vi "Multi-Device Rx Streaming Time (Four Channels) (Host).vi"() -> ()   [LabVIEW 2021]
doc: "This template is for the Simple NI-USRP Streaming design, a design that shows the basics of streaming data from an NI 294x/295x device. Refer to the block diagram for more information about how to use this template."
uses:
  SubVIs/Start Trigger.ctl
  <vilib>/userdefined/Silver/nirio_resource_slv.ctl
  <vilib>/Utility/error.llb/DialogType.ctl
  <vilib>/measure/maspectr.llb/FFT Power Spectrum and PSD for 1 Chan (CDB).vi
  <vilib>/measure/NI_MAPro.lvlib
panel:
  in  "RIO Device 1":T1="RIO1"
  in  "RIO Device 0":T1="RIO0"
  in  "config tab":T2(tab)
  in  "device 0 rx config":T4={"transfer mode"=enum."Finite", "sample rate"=10000000.0, "number of samples"=8192, "start trigger"=enum."Immediate", "daughterboard 0 config"={"rf enable 0"=TRUE, "rf config 0"={"antenna"="RX1", "frequency"=5000000000.0, "gain"=40.0}, "rf enable 1"=TRUE, "rf config 1"={"antenna"="RX2", "frequency"=5000000000.0, "gain"=40.0}, "lo configuration"=enum."Shared"}, "daughterboard 1 config"={"rf enable 2"=TRUE, "rf config 2"={"antenna"="RX1", "frequency"=5000000000.0, "gain"=40.0}, "rf enable 3"=TRUE, "rf config 3"={"antenna"="RX2", "frequency"=5000000000.0, "gain"=40.0}, "lo configuration"=enum."Shared"}} {"daughterboard 1 config"."rf config 3"."gain" format="%#.1f"; "daughterboard 1 config"."rf config 3"."frequency" format="%#.3pHz"; "daughterboard 1 config"."rf config 2"."gain" format="%#.1f"; "daughterboard 1 config"."rf config 2"."frequency" format="%#.3pHz"; "daughterboard 0 config"."rf config 1"."gain" format="%#.1f"; "daughterboard 0 config"."rf config 1"."frequency" format="%#.3pHz"; "daughterboard 0 config"."rf config 0"."gain" format="%#.1f"; "daughterboard 0 config"."rf config 0"."frequency" format="%#.3pHz"; "sample rate" format="%#.3pS/s"}
  in  "device 1 rx config":T4={"transfer mode"=enum."Finite", "sample rate"=10000000.0, "number of samples"=8192, "start trigger"=enum."Immediate", "daughterboard 0 config"={"rf enable 0"=TRUE, "rf config 0"={"antenna"="RX1", "frequency"=5000000000.0, "gain"=40.0}, "rf enable 1"=TRUE, "rf config 1"={"antenna"="RX2", "frequency"=5000000000.0, "gain"=40.0}, "lo configuration"=enum."Shared"}, "daughterboard 1 config"={"rf enable 2"=TRUE, "rf config 2"={"antenna"="RX1", "frequency"=5000000000.0, "gain"=40.0}, "rf enable 3"=TRUE, "rf config 3"={"antenna"="RX2", "frequency"=5000000000.0, "gain"=40.0}, "lo configuration"=enum."Shared"}} {"daughterboard 1 config"."rf config 3"."gain" format="%#.1f"; "daughterboard 1 config"."rf config 3"."frequency" format="%#.3pHz"; "daughterboard 1 config"."rf config 2"."gain" format="%#.1f"; "daughterboard 1 config"."rf config 2"."frequency" format="%#.3pHz"; "daughterboard 0 config"."rf config 1"."gain" format="%#.1f"; "daughterboard 0 config"."rf config 1"."frequency" format="%#.3pHz"; "daughterboard 0 config"."rf config 0"."gain" format="%#.1f"; "daughterboard 0 config"."rf config 0"."frequency" format="%#.3pHz"; "sample rate" format="%#.3pS/s"}
  out "acquiring":bool caption="Acquiring"
  in  "reference frequency source":string(combo)="REF IN" caption="Reference Frequency Source"
  in  "indicator tab":T5(tab)
  out "power spectrum":cluster{"f0":dbl, "df":dbl, "magnitude":dbl[]}[](graph) caption="Power Spectrum"
  out "iq data":waveform(dbl)[](graph) caption="I & Q Data"
  out "rx.coerced config":T6(array[cluster]) caption="Coerced Configurations" {"channel 3"."sample rate" format="%#.3pS/s"; "channel 3"."gain" format="%#_1f"; "channel 3"."if2 lo" format="%#.3pHz"; "channel 3"."if1 lo" format="%#.3pHz"; "channel 3"."frequency" format="%#.3pHz"; "channel 2"."sample rate" format="%#.3pS/s"; "channel 2"."gain" format="%#_1f"; "channel 2"."if2 lo" format="%#.3pHz"; "channel 2"."if1 lo" format="%#.3pHz"; "channel 2"."frequency" format="%#.3pHz"; "channel 1"."sample rate" format="%#.3pS/s"; "channel 1"."gain" format="%#_1f"; "channel 1"."if2 lo" format="%#.3pHz"; "channel 1"."if1 lo" format="%#.3pHz"; "channel 1"."frequency" format="%#.3pHz"; "channel 0"."sample rate" format="%#.3pS/s"; "channel 0"."gain" format="%#_1f"; "channel 0"."if2 lo" format="%#.3pHz"; "channel 0"."if1 lo" format="%#.3pHz"; "channel 0"."frequency" format="%#.3pHz"}
  in  "rx.stop":bool
  # "This template shows the basics of streaming data on multiple USRP-2945/2955 devices. Open the Project Documentation folder of the sample project and select Simple NI-USRP Streaming 2945 2955.html for information about using LO sharing with this template."
  # "Multi-Device Rx Streaming with Time"
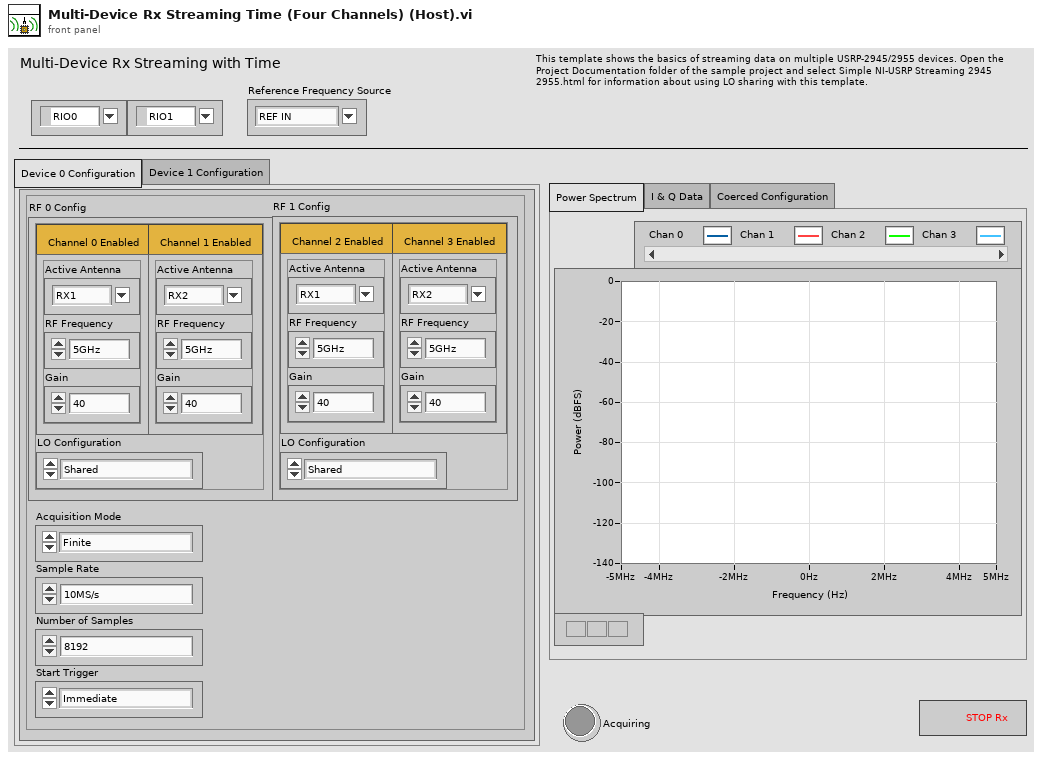
[diagram p1: front panel]
types:
  T1 = typedef "nirio_resource_slv.ctl" = tag
  T2 = enum32{"Device 0 Configuration", "Device 1 Configuration"}
  T3 = typedef "Start Trigger.ctl" = enum8{"Software", "Digital Edge", "Rx Start Trigger", "Tx Start Trigger", "Immediate", "Future Time Event"}
  T4 = cluster{"transfer mode":enum16{"Finite", "Continuous"}, "sample rate":dbl, "number of samples":u32, "start trigger":T3, "daughterboard 0 config":cluster{"rf enable 0":bool, "rf config 0":cluster{"antenna":string, "frequency":dbl, "gain":dbl}, "rf enable 1":bool, "rf config 1":cluster{"antenna":string, "frequency":dbl, "gain":dbl}, "lo configuration":enum16{"Independent", "Import", "Shared and Export", "Reimport", "Shared"}}, "daughterboard 1 config":cluster{"rf enable 2":bool, "rf config 2":cluster{"antenna":string, "frequency":dbl, "gain":dbl}, "rf enable 3":bool, "rf config 3":cluster{"antenna":string, "frequency":dbl, "gain":dbl}, "lo configuration":enum16{"Independent", "Import", "Shared and Export", "Reimport", "Shared"}}}
  T5 = enum32{"Power Spectrum", "I & Q Data", "Coerced Configuration"}
  T6 = cluster{"channel 0":cluster{"frequency":dbl, "if1 lo":dbl, "if2 lo":dbl, "gain":dbl, "sample rate":dbl}[], "channel 1":cluster{"frequency":dbl, "if1 lo":dbl, "if2 lo":dbl, "gain":dbl, "sample rate":dbl}[], "channel 2":cluster{"frequency":dbl, "if1 lo":dbl, "if2 lo":dbl, "gain":dbl, "sample rate":dbl}[], "channel 3":cluster{"frequency":dbl, "if1 lo":dbl, "if2 lo":dbl, "gain":dbl, "sample rate":dbl}[], "device id":i32}[]
  T7 = typedef "DialogType.ctl" = u16
  T8 = cluster{"transfer mode":enum16{"Finite", "Continuous"}, "sample rate":dbl, "number of samples":u32, "start trigger":T3, "daughterboard 0 config":cluster{"rf enable 0":bool, "rf config 0":cluster{"antenna":string, "frequency":dbl, "gain":dbl}, "rf enable 1":bool, "rf config 1":cluster{"antenna":string, "frequency":dbl, "gain":dbl}, "lo configuration":enum16{"Independent", "Import", "Shared and Export", "Reimport", "Shared"}}, "daughterboard 1 config":cluster{"rf enable 2":bool, "rf config 2":cluster{"antenna":string, "frequency":dbl, "gain":dbl}, "rf enable 3":bool, "rf config 3":cluster{"antenna":string, "frequency":dbl, "gain":dbl}, "lo configuration":enum16{"Independent", "Import", "Shared and Export", "Reimport", "Shared"}}}[]
  T9 = typedef "Rx Channels.ctl" = cluster{"rx config":cluster{"channel configuration":cluster{"channel enable":bool, "channel configuration":cluster{"antenna":string, "frequency":dbl, "lo frequency":dbl, "level":dbl}}[], "transfer mode":enum16{"Finite", "Continuous"}, "sample rate":dbl, "number of samples":u32, "start trigger":T3}, "reference frequency source":string, "rx.data sink":enum16{"SFP Port 0", "SFP Port 1", "Host"}, "rx.enabled channels":string[], "vertical range":dbl[], "rx.coerced configurations":cluster{"coerced frequencies":dbl[], "coerced lo frequencies":dbl[], "coerced levels":dbl[], "coerced sample rates":dbl[]}}
  T10 = typedef "niUsrpRio Config v1 Host.lvlib/niUsrpRio Session.ctl" = cluster{"FPGA Interface":refnum<k20>, "RIO Interface Number":u32, "Data Clock Rate":u32, "FPGA Data Clock Rate":u32, "Global Settings Register Bus":T11, "Radio 0 Settings Register Bus":T11, "Radio 1 Settings Register Bus":T11, "Radio Settings Bus Semaphore":T12, "DB Queues":T13[], "Characterization Data Valid?":bool, "EEPROM Header":T14, "Device Data Header":T15, "EEPROM Characterization Header":T16, "Characterization Data":T17[], "FPGA Current Version":u32, "FPGA Oldest Compatible Version":u32, "Fixed Logic Current Version":u32, "Fixed Logic Oldest Compatible Version":u32, "FPGA Radio Settings Bus Current Version":u32, "FPGA Radio Settings Bus Oldest Compatible Version":u32, "FPGA Board Config Current Version":u32, "FPGA Board Config Oldest Compatible Version":u32, "Daughterboard Clock Rate":u32, "daughterboard configuration session handles":u64[]}
  T11 = typedef "niInstr Register Bus v0 Host.lvlib/Register Bus Session.ctl" = refnum<queue>
  T12 = typedef "Semaphore RefNum" = refnum<k1>
  T13 = typedef "niUsrpRio Config v1 Host.lvlib/DB Queue Reference.ctl" = refnum<queue>
  T14 = typedef "niUsrpRio Config v1 Host.lvlib/EEPROM Header.ctl" = cluster{"Checksum":u32, "Product Code":u16, "Hardware Current Version":u16, "Hardware Oldest Compatible Version":u16, "EEPROM Map Current Version":u16, "EEPROM Map Oldest Compatible Version":u16, "User Password":string, "Pointer to Factory Header":u32, "Pointer to User Header":u32, "Recommended Interval":u16, "Number of Reserved Bytes":i32, "Number of Daughterboards":u8, "Daughterboard IDs":u16[], "Daughterboard Serial Numbers":string[]}
  T15 = typedef "niUsrpRio Config v1 Host.lvlib/EEPROM Device Data Header.ctl" = cluster{"Checksum":u32, "Number of Channels":u8, "Number of Gain Settings":u16[], "Pointer to Characterization Data":u32[], "Number of Reserved Bytes":i32, "Number of Frequencies":u16[]}
  T16 = typedef "niUsrpRio Config v1 Host.lvlib/EEPROM Characterization Header.ctl" = cluster{"Checksum":u32, "Date":timestamp, "Temperature":sgl, "Misc. Info":string, "Pointer to Device Data Header":u32, "Number of Reserved Bytes":i32}
  T17 = typedef "niUsrpRio Config v1 Host.lvlib/Characterization Data.ctl" = cluster{"Gains[dB]":dbl[], "Frequencies [Hz]":dbl[], "IQ Imbalance Table":T18[], "Measured Gains[dB]":dbl[][]}
  T18 = typedef "niUsrpRio Config v1 Host.lvlib/IQ Imbalance.ctl" = cluster{"Gain Imbalance [linear]":dbl, "Phase Imbalance [radians]":dbl, "Offset":cdb}
  T19 = cluster{"coerced frequencies":dbl[], "coerced if1 frequencies":dbl[], "coerced if2 frequencies":dbl[], "coerced gain":dbl[], "coerced sample rates":dbl[]}
  T20 = cluster{"coerced frequencies":dbl[], "coerced if1 frequencies":dbl[], "coerced if2 frequencies":dbl[], "coerced gain":dbl[], "coerced sample rates":dbl[]}[]
  T21 = cluster{"channel 0":cluster{"frequency":dbl, "if1 lo":dbl, "if2 lo":dbl, "gain":dbl, "sample rate":dbl}[], "channel 1":cluster{"frequency":dbl, "if1 lo":dbl, "if2 lo":dbl, "gain":dbl, "sample rate":dbl}[], "channel 2":cluster{"frequency":dbl, "if1 lo":dbl, "if2 lo":dbl, "gain":dbl, "sample rate":dbl}[], "channel 3":cluster{"frequency":dbl, "if1 lo":dbl, "if2 lo":dbl, "gain":dbl, "sample rate":dbl}[], "device id":i32}
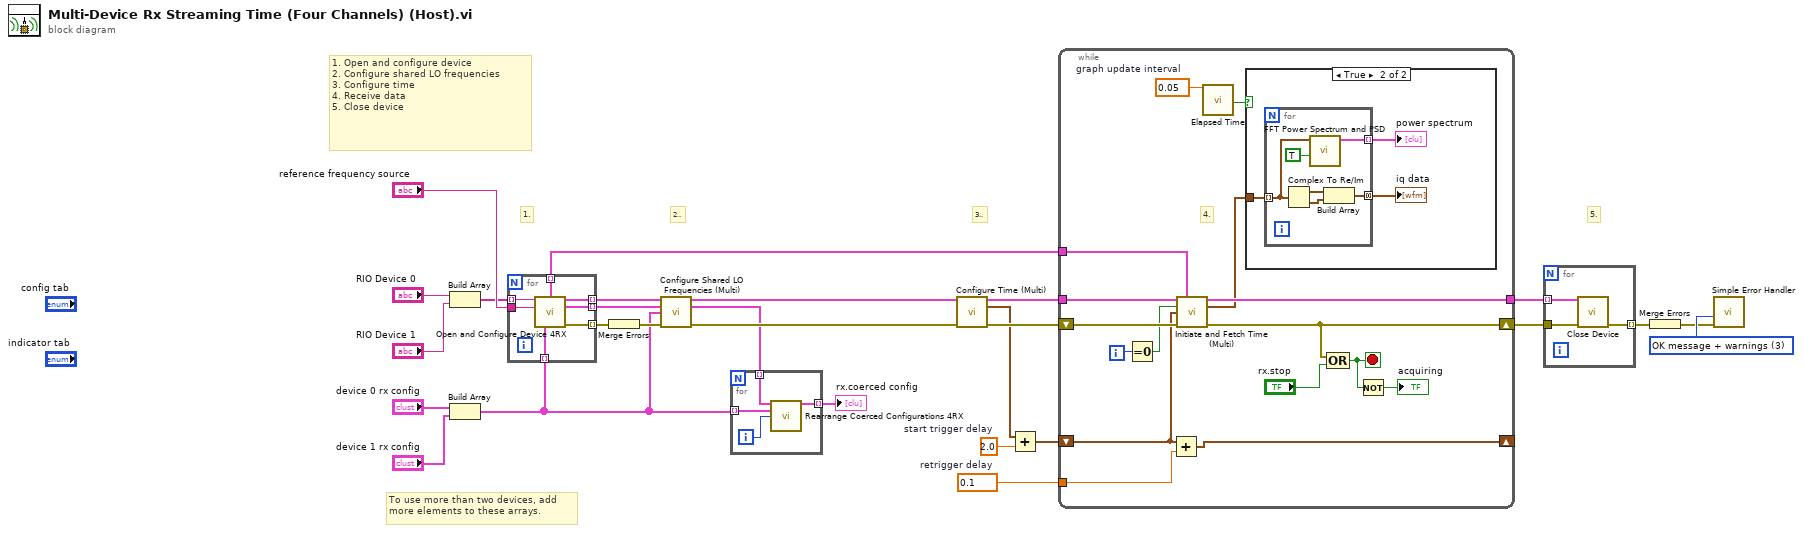
[diagram p0: block diagram]
diagram:
  w17 = 2.0  # start trigger delay
  w16 = 0.1  # retrigger delay
  w24 = T7 3 items=["no dialog", "OK message", "continue or stop message", "OK message + warnings", "continue/stop + warnings"] ("type of dialog (OK msg:1)")
  # "2.."
  # "To use more than two devices, add more elements to these arrays."
  # "5."
  # "3.."
  # "1. Open and configure device\n2. Configure shared LO frequencies\n3. Configure time\n4. Receive data\n5. Close device"
  # "1."
  n1 = Build Array("RIO Device 0", "RIO Device 1") -> (w13:T1[])
  n2 = Build Array("device 0 rx config", "device 1 rx config") -> (w3:T8)
  n3 = for {
    tunnel: [w34] -> w25 mode=indexing
    tunnel: [w33] -> w14 mode=indexing
    tunnel: "reference frequency source" -> [w32]
    tunnel: [w29] -> w7 mode=indexing
    tunnel: [w31] -> w8 mode=indexing
    tunnel: w13 -> [w30] mode=indexing
    tunnel: w3 -> [w28] mode=indexing
    n4 = call "Open and Configure Device 4RX.vi"("USRP RIO Device"=w30, "reference frequency source"=w32, "rx config"=w28) -> ("rx channels"=w33:T9, "niUsrpRio Session (out)"=w31:T10, "rx.coerced configurations"=w29:T19, "error out"=w34:errorcluster)  [unwired: 9 in]
  }
  n5 = Merge Errors(w25) -> (w4:errorcluster)
  n6 = call "Configure Shared LO Frequencies (Multi).vi"("niUsrpRio Sessions"=w8, "coerced configs"=w7, "rx configs"=w3, "error in"=w4) -> ("niUsrpRio Sessions (out)"=w6:T10[], "coerced configs out"=w2:T20, "error out"=w5:errorcluster)  [unwired: 9 in]
  n7 = for {
    tunnel: w3 -> [w38] mode=indexing
    tunnel: w2 -> [w37] mode=indexing
    tunnel: [w35] -> w1 mode=indexing
    i -> [w36]
    n8 = call "Rearrange Coerced Configurations 4RX.vi"("rx.coerced configurations"=w37, "rx config"=w38, "device id"=w36) -> ("coerced configurations"=w35:T21)  [unwired: 12 in]
  }
  "rx.coerced config" <- w1
  n9 = call "Configure Time (Multi).vi"("niUsrpRio Sessions"=w6, "error in"=w5) -> ("niUsrpRio Sessions (out)"=w21:T10[], "time"=w26:timestamp, "error out"=w27:errorcluster)  [unwired: 11 in]
  n10 = Add(x=w26, y=w17) -> (x+y=w15:timestamp)
  n11 = while {
    tunnel: w21 -> [w52]
    tunnel: [w49] -> w18
    tunnel: w14 -> [w46]
    shift-right: [w50] -> w19
    shift-left: w27 -> [w53]
    tunnel: w16 -> [w40]
    shift-right: [w39] -> _
    shift-left: w15 -> [w41]
    i -> [w51]
    stop <- w47 stop-if-true
    w45 = 0.05  # graph update interval
    # "4."
    # "Acquire and Fetch a waveform"
    n12 = Equal To 0?(x=w51) -> (x = 0?=w42:bool)
    n13 = Add(x=w41, y=w40) -> (x+y=w39:timestamp)
    n14 = call "Initiate and Fetch Time (Multi).vi"("niUsrpRio Sessions"=w52, "rx channels"=w46, "first iteration"=w42, "start trigger time"=w41, "error in"=w53) -> ("niUsrpRio Sessions (out)"=w49:T10[], "complex baseband data"=w43:waveform(cdb)[], "error out"=w50:errorcluster)  [unwired: 8 in]
    n15 = call "Elapsed Time"("Time Target (s)"=w45) -> ("Time has Elapsed"=w44:bool)  [unwired: 11 in, 7 out]
    n16 = case shown="True" w44 {
      tunnel: w43 -> [_ w57]
      frame False {
      }
      frame True {
        n17 = for {
          tunnel: [w61] -> w56 mode=concatenating
          tunnel: [w59] -> w55 mode=indexing
          tunnel: w57 -> [w60] mode=indexing
          n18 = Complex To Re/Im(x + iy=w60) -> (x=w63:waveform(dbl), y=w62:waveform(dbl))
          n19 = call-poly <vilib>:"FFT Power Spectrum and PSD.vi"("dB On (F)"=TRUE, "time signal"=w60) -> ("Power Spectrum / PSD"=w59:cluster{"f0":dbl, "df":dbl, "magnitude":dbl[]})  [unwired: 6 in, 3 out]
          n20 = Build Array(w63, w62) -> (w61:waveform(dbl)[])
        }
        "power spectrum" <- w55
        "iq data" <- w56
      }
    }
    n21 = Compound Arithmetic op=OR(w50, "rx.stop") -> (w47:bool)
    n22 = Not(x=w47) -> (.not. x?=→"acquiring":bool)
  }
  n23 = for {
    tunnel: w18 -> [w64] mode=indexing
    tunnel: w19 -> [w65]
    tunnel: [w66] -> w23 mode=indexing
    n24 = call "Close Device.vi"("niUsrpRio Session"=w64, "error in"=w65) -> ("error out"=w66:errorcluster)  [unwired: 13 in]
  }
  n25 = Merge Errors(w23) -> (w20:errorcluster)
  n26 = call <vilib>:"Simple Error Handler.vi"("type of dialog (OK msg:1)"=w24, "error in (no error)"=w20) -> ()  [unwired: 3 in, 5 out]
